vi "Circle Buffer(DBLArray).vi"(4 "reset(F)":bool, 5 "#Count":i32=1000, 6 "valid?(T)":bool=TRUE, 9 "Data":dbl[](array[numeric])) -> (3 "Array":dbl[](array[numeric]))   [LabVIEW 2017]
doc: "Maintains a circular buffer of #Count doubles that accepts an array of samples per call and returns the buffer contents."
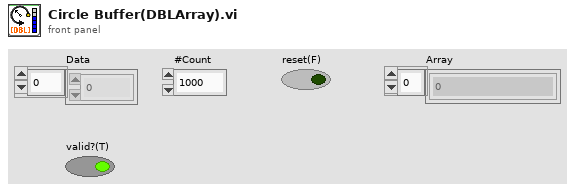
[diagram p1: front panel]
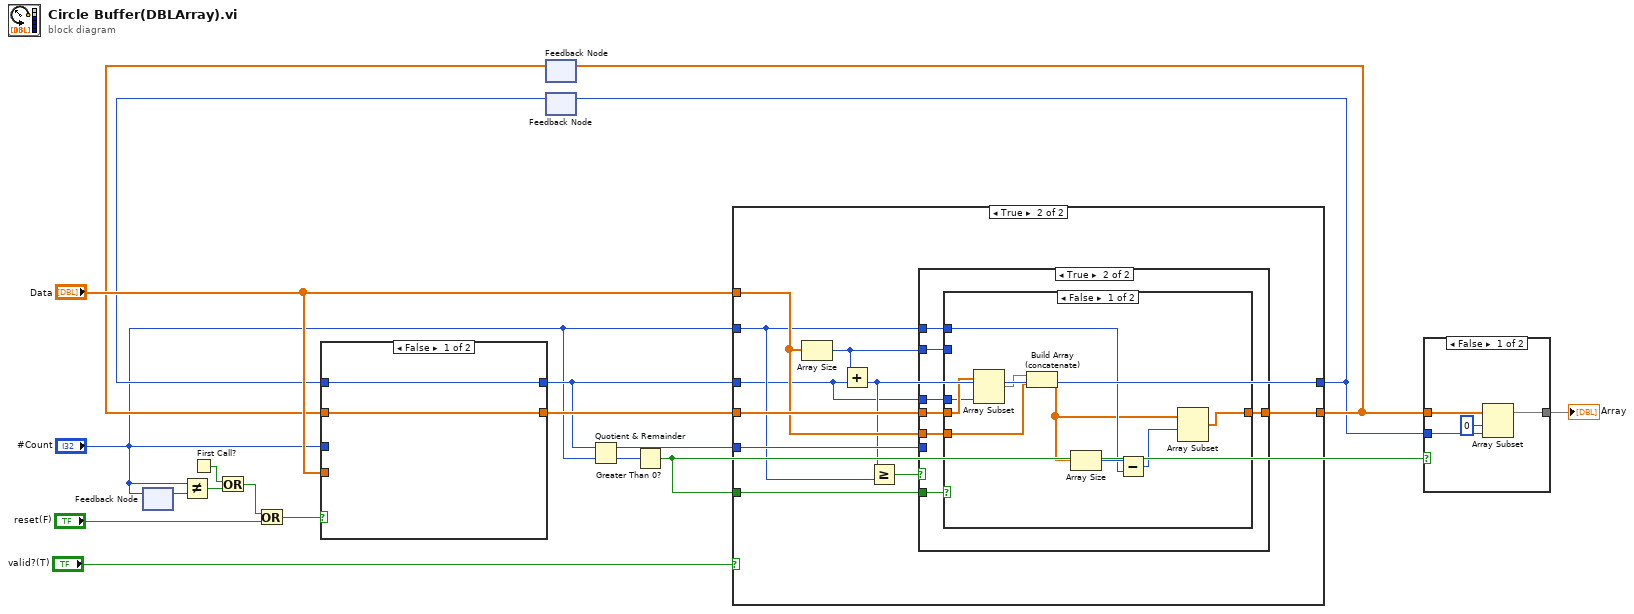
[diagram p0: block diagram]
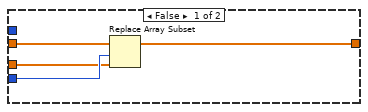
[diagram p3: hidden frame]
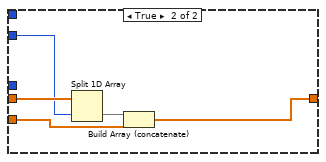
[diagram p4: hidden frame]
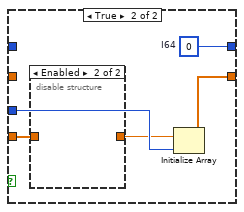
[diagram p5: hidden frame]
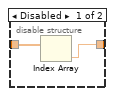
[diagram p6: hidden frame]
diagram:
  n1 = feedback #1() -> (w5:i32)  [unwired: 1 in]
  n2 = feedback-in #1("#Count") -> ()
  n3 = Not Equal?(x="#Count", y=w5) -> (x != y?=w4:bool)
  n4 = First Call?() -> (First Call?: T/F=w3:bool)
  n5 = Or(x=w3, y=w4) -> (x .or. y?=w1:bool)
  n6 = Or(x=w1, y="reset(F)") -> (x .or. y?=w9:bool)
  n7 = feedback #2() -> (w17:dbl[])  [unwired: 1 in]
  n8 = feedback #3() -> (w18:i64)  [unwired: 1 in]
  n9 = case shown="False" w9 {
    tunnel: "Data" -> [_ w24]
    tunnel: "#Count" -> [_ w26]
    tunnel: [w20 w23] -> w12
    tunnel: [w21 w22] -> w11
    tunnel: w18 -> [w21 _]
    tunnel: w17 -> [w20 _]
    frame False {
    }
    frame True {
      w22 = i64 0  # I64
      n10 = disable-structure shown="Enabled" {
        disable-tunnel: [w27 _] -> w25
        disable-tunnel: w24 -> [w28 _]
        frame Disabled {
          n11 = Index Array(array=w28) -> (element=w27:dbl)  [unwired: 1 in]
        }
        frame Enabled {
        }
      }
      n12 = Initialize Array(w25, w26) -> (w23:dbl[])
    }
  }
  n13 = Quotient & Remainder(x=w11, y="#Count") -> (x-y*floor(x/y)=w13:i64, floor(x/y)=w10:i64)
  n14 = Greater Than 0?(x=w10) -> (x > 0?=w7:bool)
  n15 = case shown="True" "valid?(T)" {
    tunnel: "Data" -> [_ w37]
    tunnel: [w29 w36] -> w6
    tunnel: [w30 w40] -> w16
    tunnel: w13 -> [_ w39]
    tunnel: w12 -> [w30 w38]
    tunnel: w11 -> [w29 w31]
    tunnel: w7 -> [_ w33]
    tunnel: "#Count" -> [_ w32]
    frame False {
    }
    frame True {
      n16 = Array Size(array=w37) -> (size(s)=w34:i32)
      n17 = Add(x=w34, y=w31) -> (x+y=w36:i64)
      n18 = Greater Or Equal?(x=w36, y=w32) -> (x >= y?=w35:bool)
      n19 = case shown="True" w35 {
        tunnel: [w44 w48] -> w40
        tunnel: w39 -> [w43 _]
        tunnel: w38 -> [w42 w51]
        tunnel: w37 -> [w41 w49]
        tunnel: w34 -> [_ w50]
        tunnel: w33 -> [_ w47]
        tunnel: w32 -> [_ w46]
        tunnel: w31 -> [_ w45]
        frame False {
          n20 = Replace Array Subset(array=w42, new element=w41, index=w43) -> (w44:dbl[])
        }
        frame True {
          n21 = case shown="False" w47 {
            tunnel: w51 -> [w54 w65]
            tunnel: w50 -> [_ w64]
            tunnel: w49 -> [w60 w62]
            tunnel: [w55 w61] -> w48
            tunnel: w46 -> [w58 _]
            tunnel: w45 -> [w52 _]
            frame False {
              n22 = Array Subset(array=w54, length=w52) -> (w53:dbl[])  [unwired: 1 in]
              n23 = Build Array (concatenate)(w53, w60) -> (w57:dbl[])
              n24 = Array Size(array=w57) -> (size(s)=w59:i32)
              n25 = Subtract(x=w59, y=w58) -> (x-y=w56:i32)
              n26 = Array Subset(array=w57, index=w56) -> (w55:dbl[])  [unwired: 1 in]
            }
            frame True {
              n27 = Split 1D Array(array=w65, index=w64) -> (second subarray=w63:dbl[])  [unwired: 1 out]
              n28 = Build Array (concatenate)(w63, w62) -> (w61:dbl[])
            }
          }
        }
      }
    }
  }
  n29 = feedback-in #2(w16) -> ()
  n30 = feedback-in #3(w6) -> ()
  n31 = case shown="False" w7 {
    tunnel: w16 -> [w69 w70]
    tunnel: w6 -> [w68 _]
    tunnel: [w66 w70] -> w15
    frame False {
      n32 = Array Subset(array=w69, index=0, length=w68) -> (w66:dbl[])
    }
    frame True {
    }
  }
  "Array" <- w15
